vi "Database New.vi"(8 "error in (no error)":errorcluster, 10 "Database File Path":path, 11 "object in":refnum<class "DatabaseAPI.lvclass">) -> (0 "error out":errorcluster, 3 "object out":refnum<class "DatabaseAPI.lvclass">)   [LabVIEW 2015, in "DatabaseAPI.lvclass"]
uses:
  DatabaseAPI.lvclass
  DatabaseAPI.lvclass/DatabaseAPI.ctl
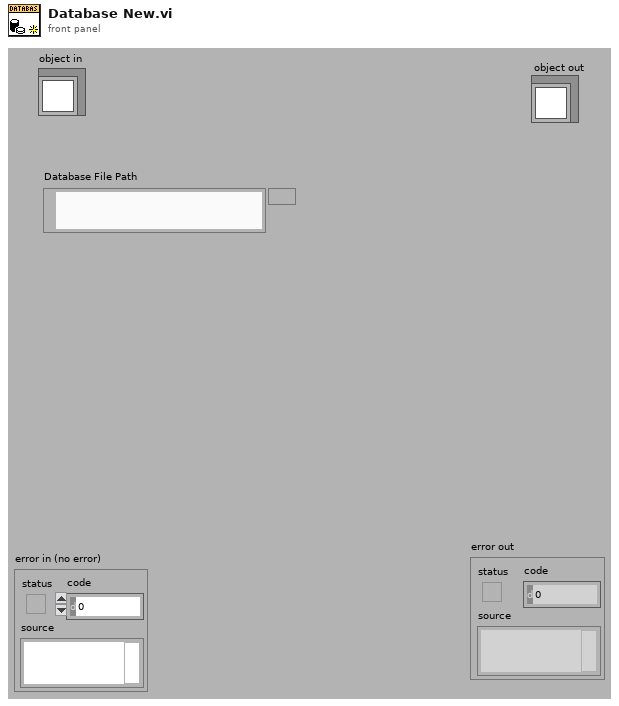
[diagram p1: front panel]
types:
  T1 = enum16{"open", "replace", "create", "open or create", "replace or create", "replace or create with confirmation"}
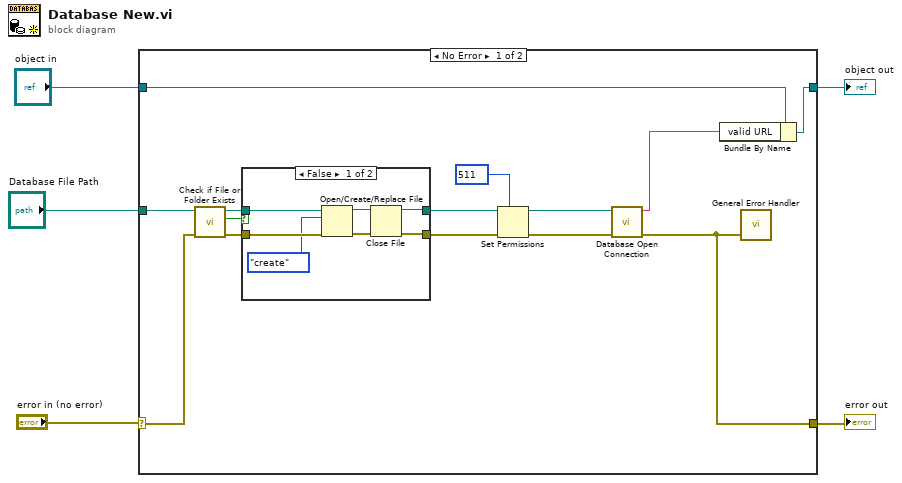
[diagram p0: block diagram]
diagram:
  n1 = case shown="No Error" "error in (no error)" {
    selector: "error in (no error)" -> [w19 w29]
    tunnel: "object in" -> [w15 w30]
    tunnel: [w13 w30] -> w4
    tunnel: [w12 w29] -> w2
    tunnel: "Database File Path" -> [w11 _]
    frame No Error {
      n2 = call <vilib>:"Check if File or Folder Exists.vi"("error in (no error)"=w19, "path"=w11) -> ("error out"=w16:errorcluster, "file or folder exists?"=w18:bool, "dup path"=w17:path)  [unwired: 7 in]
      n3 = case shown="False" w18 {
        tunnel: w17 -> [w26 w28]
        tunnel: w16 -> [w25 w27]
        tunnel: [w21 w28] -> w9
        tunnel: [w20 w27] -> w8
        frame False {
          n4 = Open/Create/Replace File(file path (use dialog)=w26, error in=w25, operation (0:open)=T1."create") -> (refnum out=w23:refnum<file>, error out=w22:errorcluster)  [unwired: 3 in, 1 out]
          n5 = Close File(refnum=w23, error in=w22) -> (path=w21:path, error out=w20:errorcluster)
        }
        frame True {
          # "It has exit!"
        }
      }
      n6 = Set Permissions(7:i16 511 ("permissions"), 8:w8, 11:w9) -> (0:w7:errorcluster, 3:w6:path)  [unwired: 2 in]
      n7 = call "Database Open Connection.vi"("error in"=w7, "Database File Path"=w6) -> ("error out"=w12:errorcluster, "valid URL"=w14:string)  [unwired: 8 in]
      n8 = Bundle By Name(cluster=w15, "valid URL"=w14) -> (w13:refnum<class "DatabaseAPI.lvclass">)
      n9 = call <vilib>:"General Error Handler.vi"("error in (no error)"=w12) -> ()  [unwired: 10 in, 5 out]
    }
    frame Error {
    }
  }
  "object out" <- w4
  "error out" <- w2
